vi "10-Tap 8-Bit Camera with DRAM (Host) - calibration.vi"() -> ()   [LabVIEW 2018]
doc: "This is the host VI for the 10-Tap 8-Bit Camera with DRAM example. This example demonstrates how to acquire images from a 10-tap, 8-bit, extended configuration, Camera Link camera and display the images on the host. This example supports area scan and line scan cameras for both continuous and finite acquisitions.\n\nThis example also demonstrates the use of DRAM as a frame buffer for very high speed acquisitions. Data packing and flow-control are also employed to maximize use of the available DRAM and FIFOs in terms of both memory space and performance.\n\nAdditionally, the example demonstrates the serial server, which allows third-party camera configuration utilities to communicate with the camera using the Camera Link serial interface while this VI is running."
uses:
  <vilib>/userdefined/High Color/nirio_resource_hc.ctl
  <vilib>/Analysis/Matrix/Datatypes/RealMatrix.ctl
  <vilib>/Platform/TimedLoop/XDataNode/timing_clust.ctl
  <vilib>/Platform/TimedLoop/XDataNode/nitl_modes.ctl
  <vilib>/Platform/TimedLoop/XDataNode/wakeup.ctl
  <vilib>/DAQmx/write.llb/DAQmx Write (Analog DBL 1Chan 1Samp).vi
  <vilib>/Analysis/baseanly.llb/Real A x B.vi
  <vilib>/FPGAPlugInAG/PCIe-1473R/niLvFpga_Open_PCIe-1473R.vi
  <vilib>/rvi/interface/common/dynamic/niFpgaDynamicAddResources.vi
  <vilib>/FPGAPlugInAG/Dynamic/niLvFpga_Reset_Dynamic.vi
  <vilib>/Analysis/Matrix/Numeric/Conversions/Array To Matrix - RA2.vi
  <userlib>/DAQNavi Polymorphic VI/create/DAQNavi Create Channel(CI-UpDown Count Value).vi
  <vilib>/Utility/error.llb/Error Cluster From Error Code.vi
  <vilib>/rvi/errors/niLvFpgaAdjustHostInterfaceError.vi
  <vilib>/FPGAPlugInAG/Dynamic/niLvFpga_Run_Dynamic.vi
  <vilib>/rvi/interface/common/niFpgaWaitOnOcc.vi
  <userlib>/DAQNavi Polymorphic VI/read/DAQNavi Read (Counter Count Value 1Chan 1Samp).vi
  <vilib>/Analysis/Matrix/Numeric/Conversions/Array To Matrix - RA.vi
  <vilib>/Analysis/Matrix/Numeric/Conversions/Matrix To Array - RM.vi
  <vilib>/DAQmx/miscellaneous.llb/DAQmx Fill In Error Info.vi
  <vilib>/FPGAPlugInAG/Dynamic/niLvFpga_Close_Dynamic.vi
  <vilib>/platform/TimedLoop/XDataNode/XDataNode.xnode
  <vilib>/rvi/interface/nirviOpenFPGA/nirviOpenFPGA.xnode
  FPGA Bitfiles/10-Tap8-bitCamer_FPGATarget_10-Tap8-bitCamer_C490DC32.lvbitx
  <vilib>/rvi/interface/nirviMethod/nirviMethod.xnode
  <vilib>/ErrorRing/Error Ring.xnode
  <vilib>/rvi/interface/nirviReadWriteControl/nirviReadWriteControl.xnode
  <vilib>/rvi/interface/nirviCloseFPGA/nirviCloseFPGA.xnode
  <vilib>/rvi/interface/Simulation/niFpgaSimulationCallBeginRW.vi
  <vilib>/rvi/errors/niLvFpgaMergeErrorWithErrorCode.vi
  NiFpgaLv.dll
  <vilib>/FPGAPlugInAG/Dynamic/niLvFpga_ConfigureFifo_Dynamic.vi
  <vilib>/FPGAPlugInAG/Dynamic/niLvFpga_StartFifo_Dynamic.vi
  <vilib>/FPGAPlugInAG/Dynamic/niLvFpga_ReadFifo_Dynamic.vi
  <vilib>/Platform/TimedLoop/XDataNode/XDNodeRunTimeDep.lvlib
  <resource>/objmgr/ni.dex.rc
  MPC_dll_4_vs17_cv3_4/x64/Release/MPC_dll_4_vs17_cv3_4.dll
  fish tracking dll vc17 opencv3_4/x64/Release/fish tracking dll vc17 opencv3_4.dll
  <vilib>/Analysis/NI_AALBase.lvlib
  <vilib>/Analysis/Matrix/NI_Matrix.lvlib
panel:
  out "Cluster":cluster{"data":i32, i32}
  out "Real Matrix 5":T1
  out "Real Matrix 4":T1
  out "Real Matrix 2":T1
  out "Real Matrix":T1
  out "A x B 2":T1
  out "A x B":T1
  out "error out":errorcluster
  in  "send":bool
  out "Is Connected":bool
  in  "update ratio":dbl
  in  "Start Serial Server":bool=TRUE
  in  "Stopped 2":bool
  in  "display":bool=TRUE
  out "Image":T2(plugin-control)
  in  "reset 2":bool
  in  "reset frame":bool
  in  "reset position":bool
  out "max load a frame":dbl
  out "max load a position":dbl
  out "# elements in queue":i32
  out "element":dbl[](array[numeric])
  in  "start sending":bool
  out "connected":bool
  in  "Acquire":bool
  out "max distance 2":i32
  out "out of FOV 2":i32
  in  "count":bool
  out "max distance":i32
  out "out of FOV":i32
  out "Stage Position Y":i32=520
  out "Stage Position X":i32=520
  out "#timeout3":i32
  out "#timeout1":i32
  out "max time4 image and position loading":dbl
  out "max time3 total":dbl
  out "max time2 detection":dbl
  out "max time1 detection+command":dbl
  out "time loading a frame":dbl
  in  "length of fish_history":i32=4
  in  "m(length of kernel)":i32=30
  out "Heading":cluster{dbl, dbl}
  out "BKG_Global":T2(plugin-control)
  out "process":i32
  in  "Target Y":i32(slide)=171 min=0 max=384 scale=130.0..230.0
  in  "Target X":i32(slide)=179 min=0 max=520 scale=130.0..230.0
  out "y":dbl
  out "x":dbl
  in  "Controller":picture
  out "Y Resolution":i32
  out "X Resolution":i32
  in  "Track":bool
  out "Frame #":i32=72
  out "电压2":dbl
  out "电压1":dbl
  out "fish FOUND":bool
  out "Centroid":cluster{"x":i32, "y":i32}
  out "TimeDelay":dbl
  in  "DMA Buffer Size\n(In Images)":u32=64 caption="DMA Buffer Size"
  in  "Signal Mapping":T3(ring)=enum."Basler 10-tap"
  out "Acq In Progress":bool
  in  "Line Scan":bool
  in  "Cancel":bool
  out "Acq'd Frame Width":u32
  in  "Stopped":bool
  in  "RIO Device":T4="RIO0"
  out "DMA Write Timeout":bool
  out "Frames Acq'd":u32
  out "Acq'd Frame Height":u32
  in  "Stop":bool
  in  "Image Height":u32=360 max=65535
  in  "Image Width":u32=360 max=65535 step=40
  out "Initialized":bool
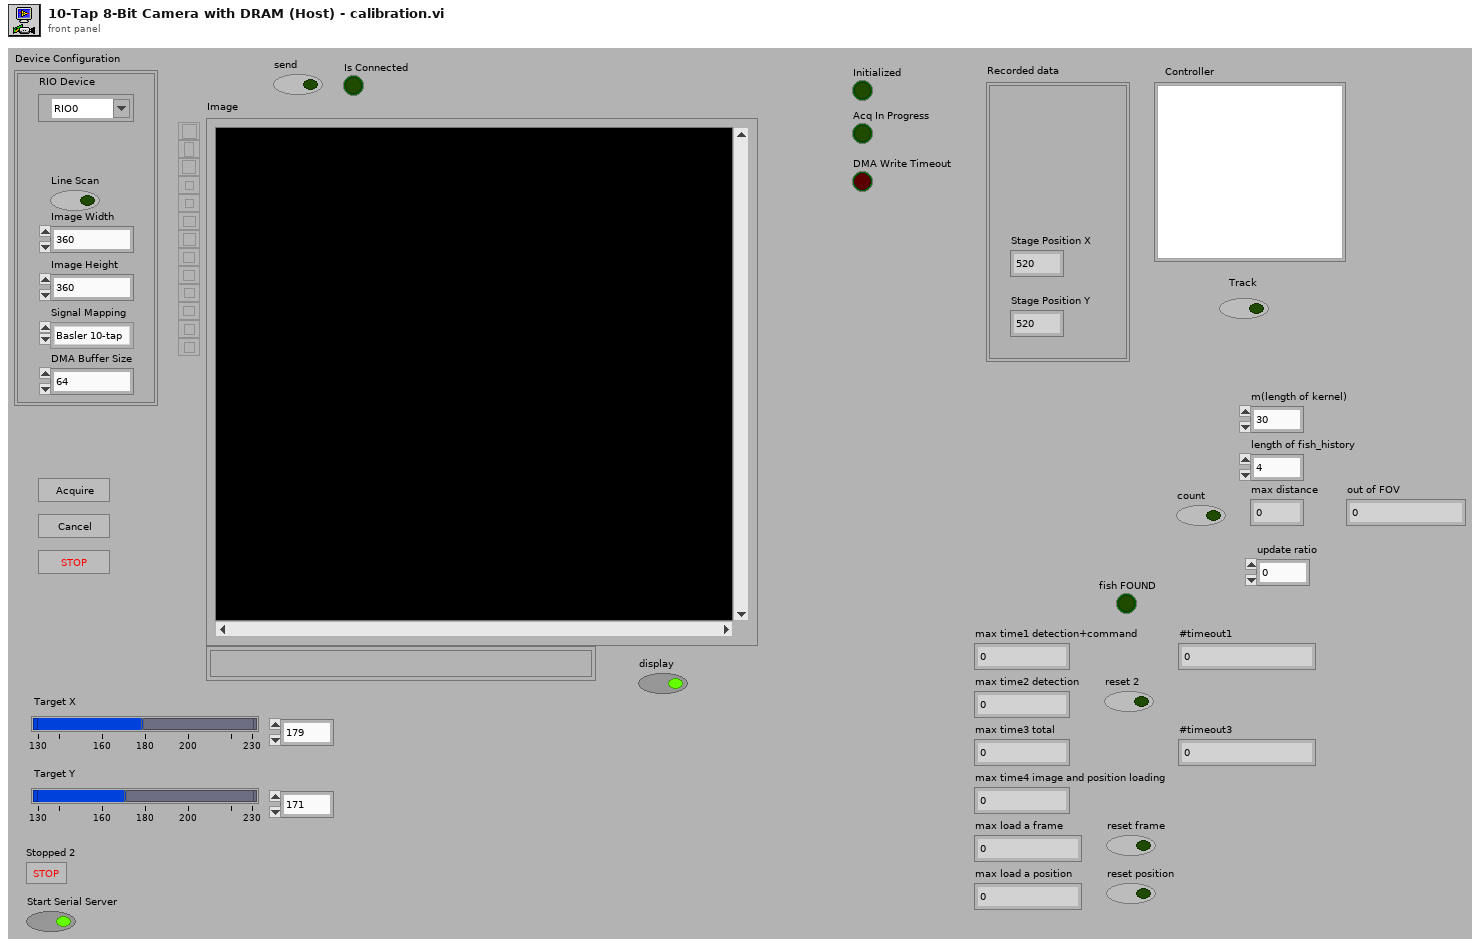
[diagram p1: front panel]
types:
  T1 = typedef "NI_Matrix.lvlib/RealMatrix.ctl" = dbl[][]
  T2 = typedef "IMAQ Image.ctl" = refnum<image>
  T3 = enum8{"Standard", "Basler 10-tap", "Vosskühler 10-tap"}
  T4 = typedef "nirio_resource_hc.ctl" = tag
  T5 = typedef "Image Type" = u32
  T6 = typedef "XDNodeRunTimeDep.lvlib/timing_clust.ctl" = cluster{"Expected End [f-1]":u64, "Actual End [f-1]":u64, "Finished Late? [f-1]":bool, "Expected End [i-1]":u64, "Actual End [i-1]":u64, "Finished Late? [i-1]":bool, "Expected Start [i]":u64, "Actual Start [i]":u64, "Expected Start [f]":u64, "Actual Start [f]":u64, "Source Name":string, "Structure Name":string, "Period":i64, "Deadline":i64, "Offset":i64, "Start":i64, "Priority":i32, "Timeout":i32, "Mode":T7, "Wakeup Reason":T8, "Error":errorcluster, "Source Type":string, "Secondary Source Type":string, "Global End Time":u64, "Global Start Time":u64, "Frame Duration":u64, "Iteration Duration":u64, "Assigned CPU":i32, "I/O Scan Engine Mode":u32}
  T7 = typedef "XDNodeRunTimeDep.lvlib/nitl_modes.ctl" = enum32{"No Change", "Process missed periods, maintain original phase", "Discard missed periods, maintain original phase", "Process missed periods, ignore original phase", "Discard missed periods, ignore original phase"}
  T8 = typedef "XDNodeRunTimeDep.lvlib/wakeup.ctl" = enum32{"Normal", "Aborted", "Asynchronous wakeup", "Timing source error", "Timed loop error", "Timeout"}
  T9 = enum16{"big-endian, network order", "native, host order", "little-endian"}
  T10 = enum32{"Map Pixel Pointer", "Unmap Pixel Pointer", "Get Pixels Infos"}
  T11 = typedef "LVPoint32TypeDef.ctl" = cluster{"Horizontal":i32, "Vertical":i32}
  T12 = typedef "LVPositionTypeDef.ctl" = cluster{"Left":i32, "Top":i32}
  T13 = typedef "LVBoundsTypeDef.ctl" = cluster{"Width":u32, "Height":u32}
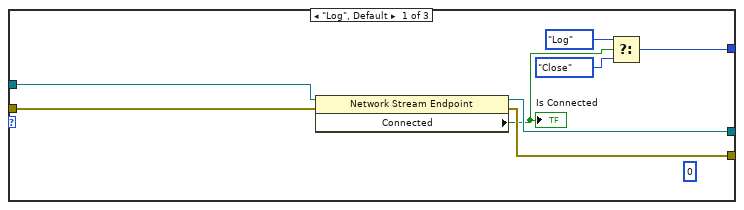
[diagram p4: hidden frame]
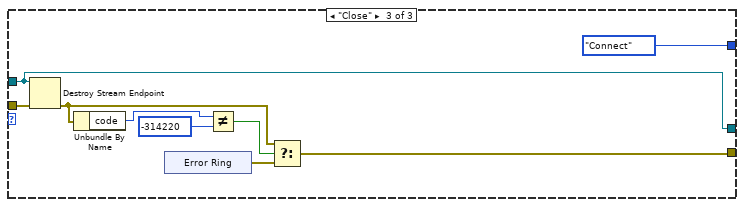
[diagram p5: hidden frame]
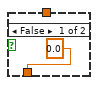
[diagram p12: hidden frame]
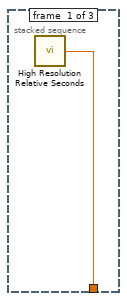
[diagram p13: hidden frame]
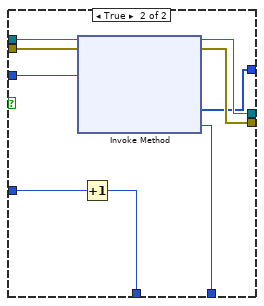
[diagram p14: hidden frame]
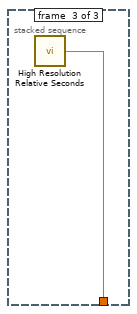
[diagram p15: hidden frame]
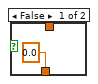
[diagram p16: hidden frame]
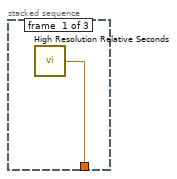
[diagram p17: hidden frame]
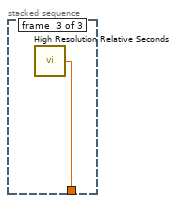
[diagram p18: hidden frame]
diagram:
  w23 = 72 ("n_templates")
  w25 = 0
  w46 = 2
  w40 = 0
  w47 = 0.0
  w72 = T5 0 items=["Grayscale (U8)", "Grayscale (I16)", "Grayscale (SGL)", "Complex (CSG)", "RGB (U32)", "HSL (U32)", "RGB (U64)", "Grayscale (U16)"] ("Image Type")
  w86 = refnum<k21> "Stage_Y"  # DAQmx任务名
  w87 = refnum<k21> "Stage_X"  # DAQmx任务名
  w89 = T5 0 items=["Grayscale (U8)", "Grayscale (I16)", "Grayscale (SGL)", "Complex (CSG)", "RGB (U32)", "HSL (U32)", "RGB (U64)", "Grayscale (U16)"] ("Image Type")
  w95 = u32 8  # Pixels per DMA word
  w126 = T5 0 items=["Grayscale (U8)", "Grayscale (I16)", "Grayscale (SGL)", "Complex (CSG)", "RGB (U32)", "HSL (U32)", "RGB (U64)", "Grayscale (U16)"] ("Image Type")
  # "Start the Serial Server to allow serial communication\nwith the camera. This allows third-party camera\nconfiguration utilites to be used."
  # "If your camera outputs active-low enable\nsignals or does not use DVAL then you \ncan change the configuration here."
  # "Configure the DMA FIFO memory buffer to be\nlarge enough for several frames. This provides\nbuffering to help deal with system latencies."
  # "Start running\nthe FPGA VI."
  # "Reset FPGA to clear\nany current state."
  # "Read the specified image\nwidth and height. In this\nexample, these must be set\nbefore starting the VI."
  # "Merge any errors.\nClean up the image.\nClose the FPGA reference.\nDisplay any errors."
  # "Acquire frames as requested.\nUse the width and height to determine how much data to read from the DMA FIFO.\nConvert the data into a Vision Image for display."
  # "Monitor the acquisition status"
  # "Create an image of the type to be displayed."
  # "Initialize the acquisition interface on the FPGA.  This will\nwait until a pixel clock is detected from the camera."
  # "Initialize the DMA FIFO for transferring\ndata from FPGA target to the host."
  # "Configure the Camera Link interface.\nThis needs to be done prior to running\nthe FPGA block diagram."
  # "Open a reference to the FPGA bitstream\nand initialize the user interface."
  n1 = flat-sequence {
    tunnel: [w132] -> w121
    tunnel: [w131] -> w130
    frame #0 {
      w135 = u32 0 ("Num Lines Acq'd")
      w134 = FALSE ("stop")
      n2 = local write "DMA Write Timeout"(w134) -> ()
      n3 = local write "Acq'd Frame Width"(w135) -> ()
      n4 = local write "Acq'd Frame Height"(w135) -> ()
      n5 = local write "Stopped"(w134) -> ()
      n6 = local write "Frames Acq'd"(w135) -> ()
      n7 = local write "Initialized"(w134) -> ()
      n8 = xnode "打开FPGA VI引用句柄"("resource name"="RIO Device") -> ("FPGA VI Reference Out"=w132:refnum<k20>, "error out"=w131:errorcluster)  [unwired: 1 in]
    }
  }
  n9 = xnode "Invoke Method"("FPGA VI Reference In"=w121, "error in"=w130) -> ("FPGA VI Reference Out"=w111:refnum<k20>, "error out"=w113:errorcluster)
  n10 = xnode "Read/Write Control"("FPGA VI Reference In"=w111, "error in"=w113, "CL Config.FVAL Active High"=TRUE ("IO Module Config.CL FVAL Active High"), "CL Config.LVAL Active High"=TRUE ("IO Module Config.CL LVAL Active High"), "CL Config.DVAL Active High"=TRUE ("IO Module Config.CL DVAL Active High"), "CL Config.Spare Active High"=TRUE ("IO Module Config.CL Spare Active High"), "CL Config.Line Scan"="Line Scan", "Acq Control.Ignore DVAL"=FALSE ("CL Config.Line Scan"), "CL Config.Configuration"=enum8{"Base", "Medium", "Full"}."Full", "CL Config.Signal Mapping"="Signal Mapping") -> ("FPGA VI Reference Out"=w114:refnum<k20>, "error out"=w112:errorcluster)
  n11 = xnode "Invoke Method"("FPGA VI Reference In"=w114, "error in"=w112) -> ("FPGA VI Reference Out"=w92:refnum<k20>, "error out"=w91:errorcluster)  [unwired: 1 in]
  n12 = Multiply(x="Image Height", y="Image Width") -> (x*y=w94:u32)
  n13 = Quotient & Remainder(x=w94, y=w95) -> (floor(x/y)=w93:u32)  [unwired: 1 out]
  n14 = Multiply(x=w93, y="DMA Buffer Size\n(In Images)") -> (x*y=w105:u32)
  n15 = xnode "Invoke Method"("FPGA VI Reference In"=w92, "error in"=w91, "请求的深度"=w105) -> ("FPGA VI Reference Out"=w120:refnum<k20>, "error out"=w119:errorcluster)  [unwired: 1 out]
  n16 = xnode "Invoke Method"("FPGA VI Reference In"=w120, "error in"=w119) -> ("FPGA VI Reference Out"=w106:refnum<k20>, "error out"=w118:errorcluster)
  n17 = xnode "读取/写入控件"("FPGA VI Reference In"=w106, "error in"=w118, "Acq Control.Initialize"=TRUE ("Arm Acquisition")) -> ("FPGA VI Reference Out"=w129:refnum<k20>, "error out"=w128:errorcluster)
  n18 = while {
    tunnel: w129 -> [w143]
    tunnel: w128 -> [w142]
    tunnel: [w141] -> w10
    tunnel: [w145] -> w102
    i -> [w137]
    stop <- w148 stop-if-true
    # "A custom error is generated if the acquisition unit has not become\ninitialized within 2 seconds. This typically occurs when a camera is\nnot connected, is not powered, or is not of the correct type."
    n19 = xnode "读取/写入控件"("FPGA VI Reference In"=w143, "error in"=w142) -> ("FPGA VI Reference Out"=w141:refnum<k20>, "error out"=w140:errorcluster, "Acq Status.Initialized"=w139:bool)
    n20 = Wait (ms)(milliseconds to wait=u32 100) -> ()  [unwired: 1 out]
    n21 = Greater?(x=w137, y=20) -> (0:w138:bool)
    n22 = case shown="True" w138 {
      tunnel: [w150 FALSE] -> w144
      tunnel: w139 -> [w150 _]
      tunnel: w140 -> [w149 w152]
      tunnel: [w149 w154] -> w145
      frame False {
      }
      frame True {
        n23 = Merge Errors(w152, errorcluster {"status"=TRUE, "code"=-8999, "source"="Acquisition Initialization: This error typically occurs when a camera is not properly connected, is not powered, or is not of the correct type."} ("error in")) -> (w154:errorcluster)
      }
    }
    "Initialized" <- w144
    n24 = Unbundle By Name(w145) -> ("status"=w147:bool)
    n25 = Or(x=w147, y=w144) -> (x .or. y?=w148:bool)
  }
  n26 = case shown="True" "Start Serial Server" {
    tunnel: [_ w155] -> w9
    tunnel: w10 -> [_ w156]
    frame False {
    }
    frame True {
      n27 = control-ref of="Stopped 2"() -> (w157:refnum<vi>)
      n28 = call "SerialServer.vi"("Stop Refnum"=w157, "FPGA VI Reference In"=w156) -> ("FPGA VI Reference Out"=w155:refnum<k20>)  [unwired: 5 in]
    }
  }
  n29 = call "IMAQ Create"("Image Name"="Image", "Image Type"=w126, "error in (no error)"=w102) -> ("New Image"=w99:T2, "error out"=w98:errorcluster)  [unwired: 2 in]
  n30 = Add(x="length of fish_history", y=1) -> (x+y=w42:i32)
  n31 = Initialize Array(0.0, 7) -> (w12:dbl[])
  n32 = Obtain Queue(max queue size (-1, unlimited)=3, name (unnamed)="tracking result" ("Image Name"), element data type=w12) -> (queue out=w8:refnum<queue>)  [unwired: 2 in, 2 out]
  n33 = Multiply(x=w46, y=w42) -> (x*y=w39:i32)
  n34 = To Unsigned Byte Integer(number=w25) -> (unsigned 8bit integer=w26:u8)
  n35 = Add(x="m(length of kernel)", y=1) -> (x+y=w27:i32)
  n36 = Initialize Array(w26, w25, w25, w25) -> (w24:u8[][][])
  n37 = for {
    N: w23 -> [_]
    shift-right: [w159] -> w22
    shift-left: w24 -> [w160]
    i -> [w158]
    w164 = T5 0 items=["Grayscale (U8)", "Grayscale (I16)", "Grayscale (SGL)", "Complex (CSG)", "RGB (U32)", "HSL (U32)", "RGB (U64)", "Grayscale (U16)"] ("Image Type")
    n38 = Number To Decimal String(number=w158) -> (decimal integer string=w168:string)  [unwired: 1 in]
    n39 = Concatenate Strings(w168, ".jpg") -> (w167:string)
    n40 = Build Path(base path=path "F:/TrackingUsingOpenCV3_with_bkg_subtr_and_pred_and_temp_matching_nodisplay - 210309/templates" ("Templates Path"), name or relative path=w167) -> (appended path=w166:path)
    n41 = call "IMAQ Create"("Image Name"="Temp", "Image Type"=w164) -> ("New Image"=w163:T2)  [unwired: 3 in, 1 out]
    n42 = call "IMAQ ReadFile"("File Path"=w166, "Image"=w163) -> ("Image Out"=w162:T2)  [unwired: 5 in, 4 out]
    n43 = call "IMAQ ImageToArray"("Image"=w162) -> ("Image Pixels (U8)"=w161:u8[][])  [unwired: 3 in, 4 out]
    n44 = Insert Into Array(array=w160, index (dim 0)=w158, new element=w161) -> (w159:u8[][][])  [unwired: 2 in]
  }
  n45 = Multiply(x=w46, y=w27) -> (x*y=w45:i32)
  n46 = Obtain Queue(max queue size (-1, unlimited)=w45, name (unnamed)="command_history", element data type=w47) -> (queue out=w49:refnum<queue>)  [unwired: 2 in, 2 out]
  n47 = Obtain Queue(max queue size (-1, unlimited)=w39, name (unnamed)="stage_position_history", element data type=w40) -> (queue out=w38:refnum<queue>)  [unwired: 2 in, 2 out]
  n48 = Obtain Queue(max queue size (-1, unlimited)=w39, name (unnamed)="fish_tr_history", element data type=w40) -> (queue out=w51:refnum<queue>)  [unwired: 2 in, 2 out]
  n49 = Obtain Queue(max queue size (-1, unlimited)=w39, name (unnamed)="fish_heading_history", element data type=w47) -> (queue out=w50:refnum<queue>)  [unwired: 2 in, 2 out]
  n50 = for "For循环" {
    N: w45 -> [_]
    tunnel: w49 -> [w173]
    tunnel: [w172] -> w48
    n51 = Lossy Enqueue Element(queue=w173, element=0.0) -> (queue out=w172:refnum<queue>)  [unwired: 1 in, 3 out]
  }
  n52 = call-poly <userlib>:"DAQNavi Create Channel.vi"("physical channels"="PCI-1784,BID#1/cntr0" ("Image Name"), "signal counting type"="AbPhaseX4" ("Image Name"), "initial value"="0" ("Image Name")) -> ("task out"=w66:i32)  [unwired: 11 in, 1 out]
  n53 = call-poly <userlib>:"DAQNavi Create Channel.vi"("physical channels"="PCI-1784,BID#1/cntr1" ("Image Name"), "signal counting type"="AbPhaseX4" ("Image Name"), "initial value"="0" ("Image Name")) -> ("task out"=w65:i32)  [unwired: 11 in, 1 out]
  n54 = call "IMAQ Create"("Image Name"="BkgImageOpenCV", "Image Type"=w72) -> ("New Image"=w74:T2)  [unwired: 3 in, 1 out]
  n55 = call <userlib>:"DAQNavi Start Task.vi"("task in"=w66) -> ("task out"=w62:i32)  [unwired: 9 in, 1 out]
  n56 = call <userlib>:"DAQNavi Start Task.vi"("task in"=w65) -> ("task out"=w61:i32)  [unwired: 9 in, 1 out]
  n57 = while "Target->Host Data Writer" {
    shift-right: [w181] -> w2
    shift-left: _ -> [w184]
    shift-right: [w180] -> _
    shift-left: _ -> [w185]
    shift-right: [w182] -> _
    shift-left: enum16{"Log", "Connect", "Close"}."Log" -> [w183]
    tunnel: w8 -> [w176]
    tunnel: [w175] -> w1
    stop <- w174 stop-if-true
    # "Send Data to Host VI"
    n58 = case shown="\"Connect\"" w183 {
      tunnel: [w202 w209 w227] -> w180
      tunnel: w185 -> [w205 _ w227]
      tunnel: w184 -> [w204 _ w228]
      tunnel: [w203 w210 w221] -> w181
      tunnel: [w206 enum16{"Log", "Connect", "Close"}."Log" enum16{"Log", "Connect", "Close"}."Connect"] -> w182
      frame "Log", Default {
        (unwired) 0 ("timeout ms")
        n59 = property class="Network Stream Endpoint"(reference=w205, error in=w204) -> (reference out=w202:refnum<k21>, error out=w203:errorcluster, "Connected"=w201:bool)
        "Is Connected" <- w201
        n60 = Select(t=enum16{"Log", "Connect", "Close"}."Log", s=w201, f=enum16{"Log", "Connect", "Close"}."Close") -> (s? t:f=w206:enum16{"Log", "Connect", "Close"})
      }
      frame "Connect" {
        n61 = Concatenate Strings("//" ("reader url"), "192.168.1.30" ("Target IP Address")) -> (w215:string)
        n62 = Concatenate Strings(w215, "/reader1" ("reader url")) -> (w213:string)
        n63 = Create Network Stream Writer Endpoint(5:-1 ("timeout in ms (-1)"), 7:70, 9:0.0, 10:w213, 11:"writer") -> (0:w210:errorcluster, 3:w209:refnum<k21>)  [unwired: 2 in]
      }
      frame "Close" {
        n64 = Destroy Stream Endpoint(8:w228, 11:w227) -> (0:w222:errorcluster)
        n65 = Unbundle By Name(w222) -> ("code"=w226:i32)
        n66 = xnode "Error Ring"() -> ("error out"=w223:errorcluster)
        n67 = Not Equal?(x=w226, y=-314220) -> (x != y?=w224:bool)
        n68 = Select(t=w222, s=w224, f=w223) -> (s? t:f=w221:errorcluster)
      }
    }
    n69 = property class="Network Stream Endpoint"(reference=w180, error in=w181) -> (reference out=w178:refnum<k21>, error out=w177:errorcluster, "Connected"=w179:bool)
    n70 = case shown="True" w179 {
      tunnel: w178 -> [_ w190]
      tunnel: w177 -> [_ w191]
      tunnel: w176 -> [w186 w189]
      tunnel: [w186 w187] -> w175
      frame False {
      }
      frame True {
        n71 = Get Queue Status(queue=w189) -> (queue out=w193:refnum<queue>)  [unwired: 2 in, 7 out]
        n72 = Dequeue Element(queue=w193) -> (queue out=w187:refnum<queue>, element=w192:dbl[])  [unwired: 2 in, 2 out]
        n73 = case shown="True" "send" {
          tunnel: w192 -> [_ w198]
          tunnel: w191 -> [_ w197]
          tunnel: w190 -> [_ w196]
          frame False {
          }
          frame True {
            w199 = 0 ("timeout ms (-1)")
            n74 = shared-variable-write(w196, w197, w198, w199) -> (w195:refnum<k21>, w200:errorcluster)  [unwired: 1 out]
            n75 = Flush Stream(8:w200, 9:w199, 11:w195) -> (0:→"error out":errorcluster)  [unwired: 1 in, 2 out]
          }
        }
      }
    }
    n76 = local read "Stop"() -> (w174:bool)
  }
  n77 = disable-structure shown="Disabled" {
    disable-tunnel: w8 -> [w231 _]
    frame Disabled {
      n78 = Concatenate Strings("//" ("reader url"), "192.168.1.19" ("Target IP Address")) -> (w242:string)
      n79 = Concatenate Strings(w242, "/reader1" ("reader url")) -> (w240:string)
      n80 = Create Network Stream Writer Endpoint(7:70, 9:0.0, 10:w240, 11:"writer") -> (0:w245:errorcluster, 3:w247:refnum<k21>)  [unwired: 3 in]
      n81 = property class="Network Stream Endpoint"(reference=w247, error in=w245) -> (reference out=w238:refnum<k21>, error out=w237:errorcluster, "Connected"=→"connected":bool)
      n82 = node-c288() -> (w251:T6)  [unwired: 4 in]
      n83 = timed-loop {
        tunnel: w231 -> [w258]
        tunnel: w238 -> [w257]
        tunnel: w237 -> [w256]
        tunnel: [w255] -> w234
        tunnel: [w254] -> w233
        tunnel: [w253] -> w232
        timing: w251 -> [_]
        timing-out: [_] -> w250
        stop <- w252 stop-if-true
        n84 = node-c288() -> ()  [unwired: 1 in, 1 out]
        n85 = case shown="True" "start sending" {
          tunnel: w257 -> [w263 w276]
          tunnel: w256 -> [w262 w275]
          tunnel: w258 -> [w264 w266]
          tunnel: [w264 w274] -> w255
          tunnel: [w263 w269] -> w254
          tunnel: [w262 w268] -> w253
          frame False {
          }
          frame True {
            w270 = 0
            n86 = Get Queue Status(queue=w266) -> (queue out=w267:refnum<queue>, # elements in queue=w265:i32)  [unwired: 2 in, 6 out]
            n87 = disable-structure shown="Disabled" {
              disable-tunnel: w265 -> [w277 _]
              frame Disabled {
                "# elements in queue" <- w277
              }
              frame Enabled {
              }
            }
            n88 = Dequeue Element(queue=w267) -> (queue out=w274:refnum<queue>, element=w273:dbl[])  [unwired: 2 in, 2 out]
            n89 = disable-structure shown="Disabled" {
              disable-tunnel: w273 -> [w278 _]
              frame Disabled {
                "element" <- w278
              }
              frame Enabled {
              }
            }
            n90 = shared-variable-write(w276, w275, w273, w270) -> (w272:refnum<k21>, w271:errorcluster)  [unwired: 1 out]
            n91 = Flush Stream(8:w271, 9:w270, 11:w272) -> (0:w268:errorcluster, 3:w269:refnum<k21>)  [unwired: 1 in, 1 out]
          }
        }
        n92 = local read "Stop"() -> (w252:bool)
        n93 = node-c288() -> ()  [unwired: 1 in, 1 out]
      }
      n94 = node-c288(w250) -> ()  [unwired: 1 out]
      n95 = Release Queue(queue=w234) -> ()  [unwired: 2 in, 3 out]
      n96 = Flush Stream(8:w232, 11:w233) -> (0:w235:errorcluster, 3:w236:refnum<k21>)  [unwired: 2 in, 1 out]
      n97 = Destroy Stream Endpoint(8:w235, 11:w236) -> ()  [unwired: 1 out]
    }
    frame Enabled {
    }
  }
  n98 = call-poly <vilib>:"Array To Matrix.vi"("Real 2D Array"=dbl[][] [[1.506559, -0.036078], [0.030048, 1.495542]]) -> ("Real Matrix"=w4:T1)
  "Real Matrix 5" <- w4
  n99 = call "IMAQ ReadFile"("File Path"=path "F:/TrackingUsingOpenCV3_with_bkg_subtr_and_pred_and_temp_matching_nodisplay/fish tracking dll vc17 opencv3_4/bkg_global.png" ("Bkg Image Path"), "Image"=w74) -> ("Image Out"=w71:T2)  [unwired: 5 in, 4 out]
  n100 = call-poly <vilib>:"Array To Matrix.vi"("Real 2D Array"=dbl[][] [[1.506559, -0.036078, 0.0], [0.030048, 1.495542, 1.506559], [-12.463135, -1.547689, 1.0]]) -> ("Real Matrix"=w5:T1)
  "Real Matrix 4" <- w5
  n101 = node-c288() -> (w17:T6)  [unwired: 4 in]
  n102 = call "IMAQ Create"("Image Name"="DstImageOpenCV", "Image Type"=w89) -> ("New Image"=w88:T2)  [unwired: 3 in, 1 out]
  n103 = while {
    tunnel: w10 -> [w291]
    tunnel: [w294] -> w115
    stop <- w293 stop-if-true
    w284 = u32 10  # Pixels per clock
    # "Update status indicators"
    n104 = Wait Until Next ms Multiple(millisecond multiple=u32 100) -> ()  [unwired: 1 out]
    n105 = xnode "Read/Write Control"("FPGA VI Reference In"=w291) -> ("error out"=w290:errorcluster, "Acq Status.Lines Per Frame"=w287:u32, "Acq Status.Frames Acq'd"=w289:u32, "Acq Status.Clocks Per Line"=w285:u32, "Acq Status.Acq In Progress"=→"Acq In Progress":bool, "Acq Status.DMA Write Timeout"=w282:bool)  [unwired: 1 in, 1 out]
    "DMA Write Timeout" <- w282
    n106 = Multiply(x=w285, y=w284) -> (x*y=w286:u32)
    n107 = disable-structure shown="Disabled" {
      disable-tunnel: w289 -> [w297 _]
      disable-tunnel: w287 -> [w296 _]
      disable-tunnel: w286 -> [w295 _]
      frame Disabled {
        "Acq'd Frame Height" <- w296
        "Frames Acq'd" <- w297
        "Acq'd Frame Width" <- w295
      }
      frame Enabled {
      }
    }
    n108 = local read "Stopped"() -> (w281:bool)
    n109 = Compound Arithmetic op=AND(w282, invert w281) -> (w283:bool)
    n110 = case shown="True" w283 {
      tunnel: w290 -> [w302 _]
      tunnel: [w302 errorcluster {"status"=TRUE, "code"=-8999, "source"="DMA Write Timeout: The write operation to the DMA FIFO on the FPGA timed out. This can be caused by the DMA FIFO not being started or the DMA FIFO overflowing. Make sure that Start is being called on the DMA FIFO. Also make sure that the host application is reading from the DMA FIFO fast enough to prevent it from overflowing."} ("error out")] -> w294
      frame False {
      }
      frame True {
      }
    }
    n111 = flat-sequence {
      tunnel: w294 -> [w301]
      tunnel: [w299] -> w293
      frame #0 {
        n112 = Unbundle By Name(w301) -> ("status"=w300:bool)
        n113 = Or(x=w300, y="Stopped") -> (x .or. y?=w299:bool)
        n114 = local write "Stopped"(w299) -> ()
      }
    }
  }
  n115 = call <vilib>:"Simple Error Handler.vi"("error in (no error)"=w2) -> ()  [unwired: 4 in, 5 out]
  n116 = Release Queue(queue=w1) -> ()  [unwired: 2 in, 3 out]
  n117 = Open/Create/Replace File(file path (use dialog)=path "E:/Time.txt" ("Folder"), operation (0:open)=4) -> (refnum out=w31:refnum<file>)  [unwired: 4 in, 2 out]
  n118 = call <vilib>:"DAQmx Start Task.vi"("task/channels in"=w86) -> ("task out"=w84:refnum<k21>)  [unwired: 13 in, 1 out]
  n119 = call <vilib>:"DAQmx Start Task.vi"("task/channels in"=w87) -> ("task out"=w85:refnum<k21>)  [unwired: 13 in, 1 out]
  n120 = timed-loop {
    tunnel: w10 -> [w427]
    tunnel: w98 -> [w426]
    tunnel: w93 -> [w323]
    tunnel: "Image Height" -> [w322]
    tunnel: "Image Width" -> [w431]
    tunnel: w99 -> [w430]
    tunnel: [w312] -> w116
    tunnel: [w429] -> w125
    tunnel: [w428] -> w123
    tunnel: w88 -> [w425]
    tunnel: w85 -> [w424]
    tunnel: w84 -> [w423]
    tunnel: [w422] -> w83
    tunnel: [w421] -> w82
    tunnel: w71 -> [w420]
    tunnel: w62 -> [w413]
    tunnel: w61 -> [w412]
    tunnel: [w411] -> w58
    tunnel: [w410] -> w57
    shift-right: [w416] -> _
    shift-left: u32 0 -> [w417]
    shift-right: [w414] -> _
    shift-left: cluster{"y":i32, "x":i32} {"y"=0, "x"=0} ("Centroid") -> [w415]
    tunnel: w48 -> [w409]
    tunnel: w51 -> [w408]
    tunnel: w50 -> [w407]
    tunnel: w38 -> [w406]
    tunnel: [w405] -> w37
    tunnel: [w404] -> w36
    tunnel: [w403] -> w35
    tunnel: [w402] -> w34
    tunnel: w31 -> [w400]
    tunnel: [w399] -> w30
    shift-right: [w398] -> _
    shift-left: _ -> [w397]
    tunnel: w23 -> [w396]
    tunnel: w22 -> [w395]
    tunnel: w8 -> [w394]
    timing: w17 -> [_]
    timing-out: [_] -> w16
    border: u32 0 -> [_]
    tunnel: w5 -> [w308]
    tunnel: w4 -> [w306]
    i -> [w401]
    stop <- w418 stop-if-true
    # "Read one frame\nfrom DMA FIFO"
    # "If we're in an acquisition, wait until\nwe have at least one frame to read."
    n121 = node-c288() -> ()  [unwired: 1 in, 1 out]
    n122 = stacked-sequence {
      tunnel: [_ w442 _] -> w429
      tunnel: w427 -> [_ w441 _]
      tunnel: w426 -> [_ w440 _]
      tunnel: [_ w439 _] -> w312
      tunnel: [_ w438 _] -> w393
      tunnel: w323 -> [_ w437 _]
      tunnel: w322 -> [_ w436 _]
      tunnel: [w435 _ _] -> w320
      tunnel: [_ _ w490] -> w321
      frame #0 {
        n123 = call <vilib>:"High Resolution Relative Seconds.vi"() -> ("relative seconds"=w435:dbl)
      }
      frame #1 {
        n124 = while {
          tunnel: [w448] -> w438
          tunnel: w437 -> [w445]
          shift-right: [w456] -> w442
          shift-left: w441 -> [w455]
          shift-right: [w449] -> w439
          shift-left: w440 -> [w454]
          tunnel: w436 -> [w443]
          stop <- w444 stop-if-true
          n125 = feedback #1() -> (w450:u32)
          n126 = while {
            tunnel: w455 -> [w486]
            tunnel: w454 -> [w485]
            tunnel: [w483] -> w453
            tunnel: [w484] -> w452
            tunnel: w450 -> [w489]
            tunnel: [w487] -> w446
            stop <- w488 stop-if-true
            n127 = xnode "Read/Write Control"("FPGA VI Reference In"=w486, "error in"=w485, "Acq Control.Cancel Acq"="Cancel") -> ("FPGA VI Reference Out"=w484:refnum<k20>, "error out"=w483:errorcluster, "Acq Status.Acq In Progress"=w482:bool, "Acq Status.Frames Acq'd"=w481:u32)
            n128 = Greater?(x=w481, y=w489) -> (0:w487:bool)
            n129 = Compound Arithmetic op=OR(invert w482, w487) -> (w488:bool)
          }
          n130 = case shown="False" w446 {
            tunnel: w445 -> [w468 w479]
            tunnel: [w463 w478] -> w456
            tunnel: w453 -> [w470 w477]
            tunnel: w452 -> [w469 w476]
            tunnel: [w457 w475] -> w451
            tunnel: w450 -> [w458 w474]
            tunnel: [w462 w473] -> w449
            tunnel: [_ w472] -> w448
            tunnel: [w468 w471] -> w447
            tunnel: w443 -> [w467 _]
            frame False {
              n131 = xnode "Read/Write Control"("FPGA VI Reference In"=w469, "error in"=w470, "Acq Control.Line Scan Height"=w467, "Acq Control.Frames To Acq"=u32 0 ("Frames To Acquire")) -> ("FPGA VI Reference Out"=w465:refnum<k20>, "error out"=w464:errorcluster)
              n132 = call "Rising Edge Detect.vi"("Input"="Acquire") -> ("Pulse"=w461:bool)  [unwired: 4 in]
              n133 = xnode "Read/Write Control"("FPGA VI Reference In"=w465, "error in"=w464, "Acq Control.Acquire"=w461) -> ("FPGA VI Reference Out"=w463:refnum<k20>, "error out"=w462:errorcluster)
              n134 = Select(t=u32 0, s="Acquire", f=w458) -> (s? t:f=w457:u32)
            }
            frame True {
              n135 = xnode "Invoke Method"("FPGA VI Reference In"=w476, "error in"=w477, "元素数量"=w479) -> ("FPGA VI Reference Out"=w478:refnum<k20>, "error out"=w473:errorcluster, "数据"=w472:u64[], "剩余元素"=w471:u32)  [unwired: 1 in]
              n136 = Increment(x=w474) -> (x+1=w475:u32)
            }
          }
          n137 = feedback-in #1(w451) -> ()
          n138 = Less?(x=w447, y=w445) -> (x < y?=w444:bool)
        }
      }
      frame #2 {
        n139 = call <vilib>:"High Resolution Relative Seconds.vi"() -> ("relative seconds"=w490:dbl)
      }
    }
    n140 = disable-structure shown="Disabled" {
      disable-tunnel: w401 -> [w432 _]
      frame Disabled {
        "process" <- w432
      }
      frame Enabled {
      }
    }
    n141 = Not(x="reset frame") -> (.not. x?=w311:bool)
    n142 = Boolean To (0,1)(Boolean=w311) -> (0, 1=w316:i16)
    n143 = Subtract(x=w321, y=w320) -> (x-y=w317:dbl)
    n144 = feedback #2(-inf) -> (w319:dbl)
    n145 = Max & Min(x=w317, y=w319) -> (max(x,y)=w314:dbl)  [unwired: 1 out]
    n146 = Multiply(x=w314, y=w316) -> (x*y=w313:dbl)
    n147 = feedback-in #2(w313) -> ()
    n148 = case shown="True" w311 {
      tunnel: w314 -> [_ w434]
      tunnel: [0.0 w434] -> w310
      frame False {
      }
      frame True {
      }
    }
    "max load a frame" <- w310
    n149 = flat-sequence {
      tunnel: w397 -> [w512]
      tunnel: w406 -> [w513]
      tunnel: w407 -> [w514]
      tunnel: w408 -> [w515]
      tunnel: w409 -> [w516]
      tunnel: w412 -> [w510]
      tunnel: w413 -> [w511]
      tunnel: w415 -> [w517]
      tunnel: w417 -> [w518]
      tunnel: w420 -> [w519]
      tunnel: w425 -> [w520]
      tunnel: w393 -> [w521]
      tunnel: w430 -> [w522]
      tunnel: w431 -> [w523]
      tunnel: w322 -> [w524]
      tunnel: [w524] -> w392
      tunnel: [w523] -> w391
      tunnel: [w522] -> w390
      tunnel: [w521] -> w389
      tunnel: [w520] -> w388
      tunnel: [w519] -> w387
      tunnel: [w518] -> w386
      tunnel: [w517] -> w385
      tunnel: [w516] -> w384
      tunnel: [w515] -> w383
      tunnel: [w514] -> w382
      tunnel: [w513] -> w381
      tunnel: [w512] -> w380
      tunnel: [w509] -> w379
      tunnel: [w508] -> w378
      tunnel: [w507] -> w377
      tunnel: [w506] -> w376
      tunnel: w396 -> [w506]
      tunnel: [w505] -> w375
      tunnel: w395 -> [w505]
      tunnel: w394 -> [w504]
      tunnel: [w504] -> w374
      tunnel: w308 -> [w492]
      tunnel: [w492] -> w307
      tunnel: w306 -> [w491]
      tunnel: [w491] -> w304
      tunnel: [w569] -> w373
      tunnel: [w568] -> w372
      tunnel: [w567] -> w371
      tunnel: [w566] -> w370
      tunnel: [w565] -> w369
      tunnel: [w564] -> w368
      tunnel: [w563] -> w367
      tunnel: [w562] -> w366
      tunnel: [w544] -> w365
      tunnel: [w542] -> w364
      tunnel: [w561] -> w363
      tunnel: [w560] -> w362
      tunnel: [w559] -> w361
      tunnel: [w558] -> w360
      tunnel: [w554] -> w359
      tunnel: [w543] -> w358
      tunnel: w392 -> [w569]
      tunnel: w391 -> [w568]
      tunnel: w390 -> [w567]
      tunnel: w389 -> [w566]
      tunnel: w388 -> [w565]
      tunnel: w387 -> [w564]
      tunnel: w386 -> [w563]
      tunnel: w385 -> [w562]
      tunnel: w384 -> [w561]
      tunnel: w383 -> [w560]
      tunnel: w382 -> [w559]
      tunnel: w381 -> [w558]
      tunnel: w380 -> [w552]
      tunnel: w379 -> [w544]
      tunnel: w378 -> [w543]
      tunnel: w377 -> [w542]
      tunnel: [w541] -> w357
      tunnel: w376 -> [w541]
      tunnel: [w540] -> w356
      tunnel: w375 -> [w540]
      tunnel: [w539] -> w355
      tunnel: w374 -> [w539]
      tunnel: [w538] -> w309
      tunnel: w307 -> [w538]
      tunnel: [w537] -> w305
      tunnel: w304 -> [w537]
      tunnel: w401 -> [w621]
      tunnel: w400 -> [w620]
      tunnel: [w619] -> w399
      tunnel: w373 -> [w670]
      tunnel: w372 -> [w669]
      tunnel: w371 -> [w668]
      tunnel: w370 -> [w666]
      tunnel: w369 -> [w571]
      tunnel: w368 -> [w641]
      tunnel: w367 -> [w638]
      tunnel: w366 -> [w595]
      tunnel: w365 -> [w614]
      tunnel: w364 -> [w613]
      tunnel: w363 -> [w632]
      tunnel: w362 -> [w631]
      tunnel: w361 -> [w630]
      tunnel: w360 -> [w629]
      tunnel: w359 -> [w617]
      tunnel: [w570] -> w354
      tunnel: [w637] -> w353
      tunnel: [w614] -> w352
      tunnel: [w613] -> w351
      tunnel: [w601] -> w350
      tunnel: [w628] -> w349
      tunnel: [w627] -> w348
      tunnel: [w626] -> w347
      tunnel: [w625] -> w346
      tunnel: [w616] -> w345
      tunnel: [w615] -> w344
      tunnel: w358 -> [w602]
      tunnel: w357 -> [w611]
      tunnel: w356 -> [w609]
      tunnel: w355 -> [w604]
      tunnel: w309 -> [w584]
      tunnel: w305 -> [w583]
      tunnel: w354 -> [w916]
      tunnel: [w916] -> w343
      tunnel: w353 -> [w915]
      tunnel: [w915] -> w342
      tunnel: w352 -> [w914]
      tunnel: [w914] -> w341
      tunnel: w351 -> [w913]
      tunnel: [w913] -> w340
      tunnel: w350 -> [w912]
      tunnel: [w912] -> w339
      tunnel: w349 -> [w911]
      tunnel: [w911] -> w338
      tunnel: w348 -> [w910]
      tunnel: [w910] -> w337
      tunnel: w347 -> [w909]
      tunnel: [w909] -> w336
      tunnel: w346 -> [w908]
      tunnel: [w908] -> w335
      tunnel: w345 -> [w907]
      tunnel: [w907] -> w334
      tunnel: w344 -> [w906]
      tunnel: [w906] -> w333
      tunnel: w343 -> [w932]
      tunnel: w342 -> [w931]
      tunnel: w341 -> [w930]
      tunnel: w340 -> [w929]
      tunnel: w339 -> [w928]
      tunnel: w338 -> [w927]
      tunnel: w337 -> [w926]
      tunnel: w336 -> [w925]
      tunnel: w335 -> [w924]
      tunnel: [w923] -> w421
      tunnel: [w922] -> w422
      tunnel: w424 -> [w921]
      tunnel: w423 -> [w920]
      tunnel: w334 -> [w919]
      tunnel: w333 -> [w918]
      tunnel: [w932] -> w332
      tunnel: [w931] -> w331
      tunnel: [w930] -> w330
      tunnel: [w929] -> w329
      tunnel: [w928] -> w328
      tunnel: [w927] -> w327
      tunnel: [w926] -> w326
      tunnel: [w925] -> w325
      tunnel: [w924] -> w324
      tunnel: [w934] -> w402
      tunnel: [w935] -> w403
      tunnel: [w936] -> w404
      tunnel: [w937] -> w405
      tunnel: [w938] -> w414
      tunnel: [w939] -> w410
      tunnel: [w940] -> w411
      tunnel: [w941] -> w416
      tunnel: [w942] -> w428
      tunnel: w332 -> [w942]
      tunnel: w331 -> [w941]
      tunnel: w330 -> [w940]
      tunnel: w329 -> [w939]
      tunnel: w328 -> [w938]
      tunnel: w327 -> [w937]
      tunnel: w326 -> [w936]
      tunnel: w325 -> [w935]
      tunnel: w324 -> [w934]
      tunnel: [w933] -> w398
      frame #0 {
        n150 = stacked-sequence {
          tunnel: w511 -> [_ w534 _]
          tunnel: w510 -> [_ w533 _]
          tunnel: [_ w532 _] -> w509
          tunnel: [_ w531 _] -> w508
          tunnel: [_ w530 _] -> w507
          tunnel: [w527 _ _] -> w503
          tunnel: [_ _ w536] -> w502
          frame #0 {
            n151 = call <vilib>:"High Resolution Relative Seconds.vi"() -> ("relative seconds"=w527:dbl)
          }
          frame #1 {
            n152 = call-poly <userlib>:"DAQNavi Read.vi"("task in"=w533) -> ("data"=w529:i32, "task out"=w530:i32)  [unwired: 9 in]
            n153 = call-poly <userlib>:"DAQNavi Read.vi"("task in"=w534) -> ("data"=w535:i32, "task out"=w532:i32)  [unwired: 9 in]
            "Stage Position X" <- w535
            n154 = Negate(x=w529) -> (-x=w528:i32)
            "Stage Position Y" <- w528
            n155 = Bundle("data"=w535, w528) -> (w531:cluster{"data":i32, i32})  [unwired: 1 in]
          }
          frame #2 {
            n156 = call <vilib>:"High Resolution Relative Seconds.vi"() -> ("relative seconds"=w536:dbl)
          }
        }
        n157 = Not(x="reset position") -> (.not. x?=w495:bool)
        n158 = Boolean To (0,1)(Boolean=w495) -> (0, 1=w497:i16)
        n159 = Subtract(x=w502, y=w503) -> (x-y=w499:dbl)
        n160 = feedback #3(-inf) -> (w501:dbl)
        n161 = Max & Min(x=w499, y=w501) -> (max(x,y)=w494:dbl)  [unwired: 1 out]
        n162 = Multiply(x=w494, y=w497) -> (x*y=w496:dbl)
        n163 = feedback-in #3(w496) -> ()
        n164 = case shown="True" w495 {
          tunnel: w494 -> [_ w526]
          tunnel: [0.0 w526] -> w493
          frame False {
          }
          frame True {
          }
        }
        "max load a position" <- w493
      }
      frame #1 {
        n165 = call <vilib>:"High Resolution Relative Seconds.vi"() -> ("relative seconds"=w554:dbl)
        n166 = feedback #4() -> (w555:dbl)  [unwired: 1 in]
        n167 = feedback-in #4(w554) -> ()
        n168 = Subtract(x=w554, y=w555) -> (x-y=w557:dbl)
        "TimeDelay" <- w557
        n169 = Greater?(x=w557, y=0.0045) -> (0:w549:bool)
        n170 = Subtract(x=w554, y=w552) -> (x-y=→"time loading a frame":dbl)
        n171 = Select(t=1, s=w549, f=0) -> (s? t:f=w546:i32)
        n172 = feedback #5(0) -> (w547:i32)
        n173 = Add(x=w546, y=w547) -> (x+y=w545:i32)
        "#timeout3" <- w545
        n174 = feedback-in #5(w545) -> ()
      }
      frame #2 {
        w648 = 30.0 ("pixel/mm")
        w633 = 0.0
        w651 = T10."Map Pixel Pointer" ("Function")
        # "Convert U64 array\nto U8 array"
        # "Convert array to\nimage for display"
        n175 = disable-structure shown="Disabled" {
          disable-tunnel: w641 -> [w681 _]
          frame Disabled {
            "BKG_Global" <- w681
          }
          frame Enabled {
          }
        }
        n176 = Add(x=1, y=w638) -> (x+y=w637:u32)
        n177 = Flatten To String(anything=w666, prepend array or string size? (T)=FALSE, byte order (0:big-endian, network order)=T9."native, host order") -> (data string=w664:string)  [unwired: 1 in, 2 out]
        n178 = disable-structure shown="Disabled" {
          disable-tunnel: w637 -> [w672 _]
          frame Disabled {
            "Frame #" <- w672
          }
          frame Enabled {
          }
        }
        n179 = String To Byte Array(string=w664) -> (unsigned byte array=w663:u8[])
        n180 = call "IMAQ GetImageSize"("Image"=w641) -> ("Y Resolution"=w639:i32, "X Resolution"=w640:i32)  [unwired: 3 in, 1 out]
        n181 = Reshape Array(w663, w670, w669) -> (w667:u8[][])
        n182 = call "IMAQ ArrayToImage"("Image Pixels (U8)"=w667, "Image"=w668) -> ("Image Out"=w570:T2)  [unwired: 8 in, 1 out]
        n183 = call "IMAQ GetImagePixelPtr"("Function"=w651, "Image"=w641) -> ("LineWidth(Pixels)"=w653:i32, "Pixel Pointer out"=w654:u64)  [unwired: 4 in, 4 out]
        n184 = expression code="atan(x)"(-0.043 ("tan(theta)")) -> (w642:dbl)
        n185 = Divide(x=w648, y=10000.0) -> (x/y=w645:dbl)
        n186 = Divide(x=w648, y=12800.0) -> (x/y=w644:dbl)
        n187 = call "IMAQ GetImageSize"("Image"=w570) -> ("Y Resolution"=w605:i32, "X Resolution"=w606:i32)  [unwired: 3 in, 1 out]
        "X Resolution" <- w606
        "Y Resolution" <- w605
        n188 = call "IMAQ GetImagePixelPtr"("Function"=w651, "Image"=w570) -> ("LineWidth(Pixels)"=w658:i32, "Pixel Pointer out"=w662:u64)  [unwired: 4 in, 4 out]
        n189 = disable-structure shown="Disabled" {
          disable-tunnel: w602 -> [w671 _]
          frame Disabled {
            "Cluster" <- w671
          }
          frame Enabled {
          }
        }
        n190 = call "IMAQ SetImageSize"("Y Resolution"=w605, "X Resolution"=w606, "Image"=w571) -> ("Image Out"=w603:T2)  [unwired: 2 in, 1 out]
        n191 = Bundle(w633, w633) -> (w608:cluster{dbl, dbl})  [unwired: 1 in]
        n192 = call "IMAQ GetImagePixelPtr"("Function"=w651, "Image"=w603) -> ("LineWidth(Pixels)"=w660:i32, "Pixel Pointer out"=w661:u64)  [unwired: 4 in, 4 out]
        n193 = dll-call lib="F:/TrackingUsingOpenCV3_with_bkg_subtr_and_pred_and_temp_matching_nodisplay - 210309/fish tracking dll vc17 opencv3_4/x64/Release/fish tracking dll vc17 opencv3_4.dll" fn="?find_centroid@@YAHPEADH0H0HHHHHPEAEHHPEAV?$Point_@H@cv@@NNNHHHHHHH22PEAV?$Point_@N@2@N@Z"("ImagePtrSrc"=w662, "LineWidthSrc"=w658, "ImagePtrDst"=w661, "LineWidthDst"=w660, "ImagePtrBkg"=w654, "LineWidthBkg"=w653, "Width"=w606, "Height"=w605, "BkgWidth"=w640, "BkgHeight"=w639, "templates"=w609, "n_templates"=w611, "TemplatesSize"=48 ("Templates size"), "position"=w602, "scale_x"=w645, "scale_y"=w644, "theta"=w642, "BinThreshold"=80, "counting_threshold"=200 ("Object Threshold"), "ROI_witdth"=110, "ROI_height"=110, "width_fish"=23, "length_fish"=115, "shift"=14, "centroid_in"=w595, "centroid_out"=w595, "heading_vector"=w608, "Update_Ratio_Bkg"="update ratio") -> ("return type"=w636:i32, "centroid_out"=w601:cluster{"y":i32, "x":i32}, "heading_vector"=w600:cluster{dbl, dbl})  [unwired: 29 in, 2 out]
        "Centroid" <- w601
        "Heading" <- w600
        n194 = Quotient & Remainder(x=w621, y=2) -> (x-y*floor(x/y)=w623:i32)  [unwired: 1 out]
        n195 = Equal To 0?(x=w636) -> (x = 0?=w607:bool)
        "fish FOUND" <- w607
        n196 = Equal?(x=w623, y=0) -> (x = y?=w593:bool)
        n197 = Unbundle(w602) -> ("data"=w599:i32, w598:i32)
        n198 = Unbundle(w600) -> (w576:dbl, w575:dbl)
        n199 = Build Array(w576, w575) -> (w574:dbl[])
        n200 = call-poly <vilib>:"Array To Matrix.vi"("Real 1D Array"=w574) -> ("Real Matrix (Column Vector)"=w573:T1)
        n201 = Transpose Matrix(1:w573) -> (0:w572:T1)
        "Real Matrix 2" <- w572
        n202 = Unbundle(w601) -> ("y"=w582:i32, "x"=w581:i32)
        n203 = Build Array(w582, w581, 1) -> (w579:i32[])
        n204 = call-poly <vilib>:"Array To Matrix.vi"("Real 1D Array"=w579) -> ("Real Matrix (Column Vector)"=w578:T1)
        n205 = Transpose Matrix(1:w578) -> (0:w577:T1)
        "Real Matrix" <- w577
        n206 = call-poly <vilib>:"A x B.vi"("B"=w584, "A"=w577) -> ("A x B"=w592:T1)  [unwired: 1 out]
        "A x B" <- w592
        n207 = call-poly <vilib>:"A x B.vi"("B"=w583, "A"=w572) -> ("A x B"=w587:T1)  [unwired: 1 out]
        "A x B 2" <- w587
        n208 = call-poly <vilib>:"Matrix To Array.vi"("Real Matrix"=w592) -> ("Real 2D Array"=w591:dbl[][])
        n209 = call-poly <vilib>:"Matrix To Array.vi"("Real Matrix"=w587) -> ("Real 2D Array"=w589:dbl[][])
        n210 = Reshape Array(w591, 2) -> (w586:dbl[])
        n211 = Reshape Array(w589, 2) -> (w585:dbl[])
        n212 = Build Array (concatenate)(w599, w598, w586, w585) -> (w597:dbl[])
        n213 = case shown="True" w593 {
          tunnel: [w673 w677] -> w618
          tunnel: w604 -> [_ w679]
          tunnel: w597 -> [_ w678]
          tunnel: w570 -> [_ w675]
          frame False {
            n214 = call <vilib>:"High Resolution Relative Seconds.vi"() -> ("relative seconds"=w673:dbl)
          }
          frame True {
            n215 = call <vilib>:"High Resolution Relative Seconds.vi"() -> ("relative seconds"=w677:dbl)
            n216 = Build Array (concatenate)(w677, w678) -> (w676:dbl[])
            n217 = case shown="True" "display" {
              tunnel: w675 -> [_ w680]
              frame False {
              }
              frame True {
                "Image" <- w680
              }
            }
            n218 = Lossy Enqueue Element(queue=w679, element=w676) -> ()  [unwired: 1 in, 4 out]
          }
        }
        n219 = And(x=w607, y="Track") -> (x .and. y?=w596:bool)
        n220 = case shown="True" w596 {
          tunnel: [w693 w751] -> w616
          tunnel: [w694 w752] -> w615
          tunnel: w632 -> [w684 w818]
          tunnel: w631 -> [w691 w817]
          tunnel: w630 -> [w689 w816]
          tunnel: w582 -> [_ w737]
          tunnel: w581 -> [_ w738]
          tunnel: w576 -> [_ w808]
          tunnel: w575 -> [_ w807]
          tunnel: w629 -> [w687 w801]
          tunnel: w599 -> [_ w799]
          tunnel: w598 -> [_ w798]
          tunnel: [w685 w777] -> w628
          tunnel: [w686 w782] -> w627
          tunnel: [w690 w781] -> w626
          tunnel: [w688 w780] -> w625
          tunnel: w617 -> [_ w757]
          tunnel: w620 -> [w692 w756]
          tunnel: [w692 w755] -> w619
          tunnel: w618 -> [_ w753]
          frame False {
            n221 = event shown="[1] \"Controller\": Mouse Down" {
              selector: _ -> [_ _ _]
              dyn-events: _ -> [_ _ _]
              timeout: 1 -> [_ _ _]
              event "Controller": Mouse Up {
                n222 = event-data() -> ()  [unwired: 1 in, 8 out]
                n223 = local write "x"(0.0) -> ()
                n224 = local write "y"(0.0) -> ()
              }
              event "Controller": Mouse Down {
                n225 = event-data() -> ("Coords"=w721:T11)  [unwired: 1 in, 7 out]
                n226 = property on="Controller" class="Pict"() -> ("Position"=w720:T12, "Bounds"=w715:T13)  [unwired: 2 in, 2 out]
                n227 = Unbundle By Name(w721) -> ("Horizontal"=w719:i32, "Vertical"=w717:i32)
                n228 = Unbundle By Name(w715) -> ("Width"=w713:u32, "Height"=w709:u32)
                n229 = Unbundle By Name(w720) -> ("Left"=w718:i32, "Top"=w716:i32)
                n230 = Subtract(x=w717, y=w716) -> (x-y=w710:i32)
                n231 = Subtract(x=w719, y=w718) -> (x-y=w714:i32)
                n232 = Divide(x=w710, y=w709) -> (x/y=w702:dbl)
                n233 = Divide(x=w714, y=w713) -> (x/y=w712:dbl)
                n234 = Subtract(x=w702, y=0.5) -> (x-y=w705:dbl)
                n235 = Subtract(x=w712, y=0.5) -> (x-y=w706:dbl)
                n236 = Multiply(x=w706, y=-5.0) -> (x*y=→"x":dbl)
                n237 = Multiply(x=w705, y=5.0) -> (x*y=→"y":dbl)
              }
              event Timeout {
                n238 = event-data() -> ()  [unwired: 1 in, 3 out]
              }
            }
            n239 = Get Queue Status(queue=w684) -> (queue out=w683:refnum<queue>, max queue size=w682:i32)  [unwired: 2 in, 6 out]
            n240 = for "For循环" {
              N: w682 -> [_]
              tunnel: w683 -> [w698]
              tunnel: [w697] -> w685
              n241 = Lossy Enqueue Element(queue=w698, element=0.0) -> (queue out=w697:refnum<queue>)  [unwired: 1 in, 3 out]
            }
            n242 = Flush Queue(queue=w691) -> (queue out=w690:refnum<queue>)  [unwired: 1 in, 2 out]
            n243 = Flush Queue(queue=w689) -> (queue out=w688:refnum<queue>)  [unwired: 1 in, 2 out]
            n244 = Flush Queue(queue=w687) -> (queue out=w686:refnum<queue>)  [unwired: 1 in, 2 out]
            n245 = local read "y"() -> (w694:dbl)
            n246 = local read "x"() -> (w693:dbl)
          }
          frame True {
            w742 = 0
            w749 = 23
            w762 = 0.0
            w771 = 2
            w775 = TRUE
            w787 = 1.0
            n247 = local read "Target Y"() -> (w739:i32)
            n248 = Subtract(x=w738, y=w739) -> (x-y=w733:i32)
            n249 = Absolute Value(x=w733) -> (abs(x)=w732:i32)
            n250 = Bundle("Target X"="Target X", "Target Y"="Target Y") -> (w758:cluster{"Target X":i32, "Target Y":i32})  [unwired: 1 in]
            n251 = Greater?(x=w732, y=w749) -> (0:w747:bool)
            n252 = local read "Target X"() -> (w736:i32)
            n253 = Get Queue Status(queue=w818, return elements? (F)=w775) -> (queue out=w778:refnum<queue>, elements=w766:dbl[])  [unwired: 1 in, 6 out]
            n254 = Subtract(x=w737, y=w736) -> (x-y=w731:i32)
            n255 = Get Queue Status(queue=w817) -> (queue out=w812:refnum<queue>, max queue size=w769:i32, # elements in queue=w813:i32)  [unwired: 2 in, 5 out]
            n256 = Equal?(x=w813, y=0) -> (x = y?=w814:bool)
            n257 = Absolute Value(x=w731) -> (abs(x)=w730:i32)
            n258 = Quotient & Remainder(x=w769, y=2) -> (floor(x/y)=w767:i32)  [unwired: 1 out]
            n259 = case shown="True" w814 {
              tunnel: w812 -> [w895 w898]
              tunnel: w737 -> [w894 w899]
              tunnel: w767 -> [_ w900]
              tunnel: [w891 w897] -> w811
              tunnel: w738 -> [w893 w896]
              frame False {
                n260 = Lossy Enqueue Element(queue=w895, element=w894) -> (queue out=w892:refnum<queue>)  [unwired: 1 in, 3 out]
                n261 = Lossy Enqueue Element(queue=w892, element=w893) -> (queue out=w891:refnum<queue>)  [unwired: 1 in, 3 out]
              }
              frame True {
                n262 = for "For循环" {
                  N: w900 -> [_]
                  tunnel: w899 -> [w905]
                  tunnel: w898 -> [w904]
                  tunnel: [w901] -> w897
                  tunnel: w896 -> [w902]
                  n263 = Lossy Enqueue Element(queue=w904, element=w905) -> (queue out=w903:refnum<queue>)  [unwired: 1 in, 3 out]
                  n264 = Lossy Enqueue Element(queue=w903, element=w902) -> (queue out=w901:refnum<queue>)  [unwired: 1 in, 3 out]
                }
              }
            }
            n265 = Get Queue Status(queue=w811, return elements? (F)=w775) -> (queue out=w781:refnum<queue>, elements=w776:i32[])  [unwired: 1 in, 6 out]
            n266 = Greater?(x=w730, y=w749) -> (0:w748:bool)
            n267 = Or(x=w747, y=w748) -> (x .or. y?=w746:bool)
            n268 = Get Queue Status(queue=w816) -> (queue out=w805:refnum<queue>, max queue size=w772:i32, # elements in queue=w809:i32)  [unwired: 2 in, 5 out]
            n269 = Equal?(x=w809, y=0) -> (x = y?=w806:bool)
            n270 = Select(t=1, s=w746, f=w742) -> (s? t:f=w744:i32)
            n271 = Quotient & Remainder(x=w772, y=w771) -> (floor(x/y)=w770:i32)  [unwired: 1 out]
            n272 = case shown="True" w806 {
              tunnel: w805 -> [w880 w883]
              tunnel: w808 -> [w879 w884]
              tunnel: w770 -> [_ w885]
              tunnel: [w876 w882] -> w804
              tunnel: w807 -> [w878 w881]
              frame False {
                n273 = Lossy Enqueue Element(queue=w880, element=w879) -> (queue out=w877:refnum<queue>)  [unwired: 1 in, 3 out]
                n274 = Lossy Enqueue Element(queue=w877, element=w878) -> (queue out=w876:refnum<queue>)  [unwired: 1 in, 3 out]
              }
              frame True {
                n275 = for "For循环" {
                  N: w885 -> [_]
                  tunnel: w884 -> [w890]
                  tunnel: w883 -> [w889]
                  tunnel: [w887] -> w882
                  tunnel: w881 -> [w886]
                  n276 = Lossy Enqueue Element(queue=w889, element=w890) -> (queue out=w888:refnum<queue>)  [unwired: 1 in, 3 out]
                  n277 = Lossy Enqueue Element(queue=w888, element=w886) -> (queue out=w887:refnum<queue>)  [unwired: 1 in, 3 out]
                }
              }
            }
            n278 = Get Queue Status(queue=w804, return elements? (F)=w775) -> (queue out=w780:refnum<queue>, elements=w764:dbl[])  [unwired: 1 in, 6 out]
            n279 = local read "m(length of kernel)"() -> (w796:i32)
            n280 = local read "length of fish_history"() -> (w794:i32)
            n281 = feedback #6(w742) -> (w728:i32)
            n282 = expression code="atan(x)"(-0.043) -> (w788:dbl)
            n283 = Divide(x=1.0, y=30.0) -> (x/y=w789:dbl)
            n284 = Get Queue Status(queue=w801) -> (queue out=w800:refnum<queue>, max queue size=w774:i32, # elements in queue=w802:i32)  [unwired: 2 in, 5 out]
            n285 = Quotient & Remainder(x=w774, y=w771) -> (floor(x/y)=w773:i32)  [unwired: 1 out]
            n286 = Equal?(x=w802, y=0) -> (x = y?=w754:bool)
            n287 = case shown="True" w754 {
              tunnel: w800 -> [w865 w868]
              tunnel: w799 -> [w864 w869]
              tunnel: w773 -> [_ w870]
              tunnel: [w861 w867] -> w797
              tunnel: w798 -> [w863 w866]
              frame False {
                n288 = Lossy Enqueue Element(queue=w865, element=w864) -> (queue out=w862:refnum<queue>)  [unwired: 1 in, 3 out]
                n289 = Lossy Enqueue Element(queue=w862, element=w863) -> (queue out=w861:refnum<queue>)  [unwired: 1 in, 3 out]
              }
              frame True {
                n290 = for "For循环" {
                  N: w870 -> [_]
                  tunnel: w869 -> [w875]
                  tunnel: w868 -> [w874]
                  tunnel: [w871] -> w867
                  tunnel: w866 -> [w872]
                  n291 = Lossy Enqueue Element(queue=w874, element=w875) -> (queue out=w873:refnum<queue>)  [unwired: 1 in, 3 out]
                  n292 = Lossy Enqueue Element(queue=w873, element=w872) -> (queue out=w871:refnum<queue>)  [unwired: 1 in, 3 out]
                }
              }
            }
            n293 = Get Queue Status(queue=w797, return elements? (F)=w775) -> (queue out=w782:refnum<queue>, elements=w765:i32[])  [unwired: 1 in, 6 out]
            n294 = Max & Min(x=w730, y=w732) -> (max(x,y)=w741:i32)  [unwired: 1 out]
            n295 = Divide(x=w787, y=10000.0) -> (x/y=w784:dbl)
            n296 = Divide(x=w787, y=12800.0) -> (x/y=w783:dbl)
            n297 = feedback #7(w742) -> (w734:i32)
            n298 = case shown="True" "count" {
              tunnel: [w819 w821] -> w735
              tunnel: w734 -> [_ w820]
              tunnel: w728 -> [_ w821]
              tunnel: [w819 w820] -> w727
              frame False {
                w819 = 0
                "out of FOV 2" <- w819
                "max distance 2" <- w819
              }
              frame True {
                "out of FOV" <- w821
                "max distance" <- w820
              }
            }
            n299 = Add(x=w735, y=w744) -> (x+y=w743:i32)
            n300 = feedback-in #6(w743) -> ()
            n301 = Max & Min(x=w741, y=w727) -> (max(x,y)=w740:i32)  [unwired: 1 out]
            n302 = feedback-in #7(w740) -> ()
            n303 = Bundle(w762, w762) -> (w761:cluster{dbl, dbl})  [unwired: 1 in]
            n304 = dll-call lib="F:/TrackingUsingOpenCV3_with_bkg_subtr_and_pred_and_temp_matching_nodisplay - 210309/MPC_dll_4_vs17_cv3_4/x64/Release/MPC_dll_4_vs17_cv3_4.dll" fn="?MPC_dll@@YAHHHHNNNHNNNNNPEAV?$Point_@H@cv@@PEANPEAH21PEAV?$Point_@N@2@@Z"("m"=w796, "predict_length"=6 ("predict length"), "fish_history_length"=w794, "gammaX"=0.06, "gammaY"=0.06, "max_command"=10.0, "shift_head2yolk"=22, "scale_x"=w789, "scale_y"=w789, "theta"=w788, "scale_x2"=w784, "scale_y2"=w783, "dst_fish_position"=w758, "command_history_array"=w766, "position_history_array"=w765, "fish_tr_history_c_array"=w776, "fish_direction_history_c_array"=w764, "c0"=w761) -> ("return type"=w726:i32, "c0"=w763:cluster{dbl, dbl})  [unwired: 20 in, 2 out]
            n305 = Equal To 0?(x=w726) -> (x = 0?=w724:bool)
            n306 = Not(x=w724) -> (.not. x?=w725:bool)
            n307 = case shown="False" w725 {
              tunnel: w757 -> [w848 w860]
              tunnel: w756 -> [w847 w859]
              tunnel: [w847 w858] -> w755
              tunnel: w753 -> [w849 w857]
              frame False {
                w837 = -inf
                n308 = local read "time loading a frame"() -> (w840:dbl)
                n309 = local read "TimeDelay"() -> (w842:dbl)
                n310 = call <vilib>:"High Resolution Relative Seconds.vi"() -> ("relative seconds"=w850:dbl)
                n311 = Not(x="reset 2") -> (.not. x?=w826:bool)
                n312 = Boolean To (0,1)(Boolean=w826) -> (0, 1=w825:i16)
                n313 = Subtract(x=w850, y=w848) -> (x-y=w827:dbl)
                n314 = Subtract(x=w849, y=w848) -> (x-y=w844:dbl)
                n315 = feedback #8(w837) -> (w846:dbl)
                n316 = feedback #9(w837) -> (w843:dbl)
                n317 = feedback #10(w837) -> (w845:dbl)
                n318 = Max & Min(x=w827, y=w846) -> (max(x,y)=w836:dbl)  [unwired: 1 out]
                "max time1 detection+command" <- w836
                n319 = feedback-in #8(w836) -> ()
                n320 = Max & Min(x=w842, y=w843) -> (max(x,y)=w839:dbl)  [unwired: 1 out]
                "max time3 total" <- w839
                n321 = feedback-in #9(w839) -> ()
                n322 = Max & Min(x=w844, y=w845) -> (max(x,y)=w824:dbl)  [unwired: 1 out]
                "max time2 detection" <- w824
                n323 = Multiply(x=w824, y=w825) -> (x*y=w823:dbl)
                n324 = feedback-in #10(w823) -> ()
                n325 = Greater?(x=w827, y=0.003) -> (0:w834:bool)
                n326 = feedback #11(w837) -> (w841:dbl)
                n327 = Select(t=1, s=w834, f=0) -> (s? t:f=w831:i32)
                n328 = Max & Min(x=w840, y=w841) -> (max(x,y)=w838:dbl)  [unwired: 1 out]
                "max time4 image and position loading" <- w838
                n329 = feedback-in #11(w838) -> ()
                n330 = feedback #12(0) -> (w830:i32)
                n331 = Add(x=w831, y=w830) -> (x+y=w829:i32)
                "#timeout1" <- w829
                n332 = feedback-in #12(w829) -> ()
              }
              frame True {
                n333 = call <vilib>:"High Resolution Relative Seconds.vi"() -> ("relative seconds"=w856:dbl)
                n334 = local read "TimeDelay"() -> (w854:dbl)
                n335 = local read "time loading a frame"() -> (w851:dbl)
                n336 = Subtract(x=w856, y=w860) -> (x-y=w855:dbl)
                n337 = Subtract(x=w857, y=w860) -> (x-y=w853:dbl)
                n338 = Format Into String(initial string=w859, w855, w853, w854, w851, "\r") -> (resulting string=w858:refnum<file>)  [unwired: 2 in, 1 out]
              }
            }
            n339 = Unbundle(w763) -> (w751:dbl, w752:dbl)
            n340 = Lossy Enqueue Element(queue=w778, element=w751) -> (queue out=w779:refnum<queue>)  [unwired: 1 in, 3 out]
            n341 = Lossy Enqueue Element(queue=w779, element=w752) -> (queue out=w777:refnum<queue>)  [unwired: 1 in, 3 out]
          }
        }
      }
      frame #3 {
      }
      frame #4 {
        n342 = Negate(x=w918) -> (-x=w917:dbl)
        "电压2" <- w917
        n343 = call-poly <vilib>:"DAQmx Write.vi"("task/channels in"=w921, "data"=w919) -> ("task out"=w922:refnum<k21>)  [unwired: 11 in, 2 out]
        n344 = call-poly <vilib>:"DAQmx Write.vi"("task/channels in"=w920, "data"=w917) -> ("task out"=w923:refnum<k21>)  [unwired: 11 in, 2 out]
        "电压1" <- w919
      }
      frame #5 {
        n345 = call <vilib>:"High Resolution Relative Seconds.vi"() -> ("relative seconds"=w933:dbl)
      }
    }
    n346 = flat-sequence {
      tunnel: w312 -> [w947]
      tunnel: [w945] -> w419
      frame #0 {
        n347 = Unbundle By Name(w947) -> ("status"=w948:bool)
        n348 = local read "Stopped"() -> (w946:bool)
        n349 = Compound Arithmetic op=OR(w948, "Stop", w946) -> (w945:bool)
        n350 = local write "Stopped"(w945) -> ()
      }
    }
    n351 = feedback-in #13(w419) -> ()
    n352 = feedback #13() -> (w418:bool)  [unwired: 1 in]
    n353 = node-c288() -> ()  [unwired: 1 in, 1 out]
  }
  n354 = Close File(refnum=w30) -> ()  [unwired: 1 in, 2 out]
  n355 = call-poly <vilib>:"DAQmx Write.vi"("task/channels in"=w83, "data"=0.0) -> ("task out"=w81:refnum<k21>)  [unwired: 11 in, 2 out]
  n356 = call <vilib>:"DAQmx Stop Task.vi"("task/channels in"=w81) -> ("task out"=w77:refnum<k21>)  [unwired: 13 in, 1 out]
  n357 = call-poly <vilib>:"DAQmx Write.vi"("task/channels in"=w82, "data"=0.0) -> ("task out"=w79:refnum<k21>)  [unwired: 11 in, 2 out]
  n358 = call <vilib>:"DAQmx Stop Task.vi"("task/channels in"=w79) -> ("task out"=w76:refnum<k21>)  [unwired: 13 in, 1 out]
  n359 = call <vilib>:"DAQmx Clear Task.vi"("task in"=w77) -> ()  [unwired: 14 in, 1 out]
  n360 = call <vilib>:"DAQmx Clear Task.vi"("task in"=w76) -> ()  [unwired: 14 in, 1 out]
  n361 = node-c288(w16) -> ()  [unwired: 1 out]
  n362 = Release Queue(queue=w37) -> ()  [unwired: 2 in, 3 out]
  n363 = Release Queue(queue=w36) -> ()  [unwired: 2 in, 3 out]
  n364 = Release Queue(queue=w35) -> ()  [unwired: 2 in, 3 out]
  n365 = Release Queue(queue=w34) -> ()  [unwired: 2 in, 3 out]
  n366 = call <userlib>:"DAQNavi Stop Task.vi"("task in"=w58) -> ("task out"=w60:i32)  [unwired: 1 in, 1 out]
  n367 = Merge Errors(w116, w115) -> (w117:errorcluster)
  n368 = call <userlib>:"DAQNavi Stop Task.vi"("task in"=w57) -> ("task out"=w59:i32)  [unwired: 1 in, 1 out]
  n369 = flat-sequence {
    tunnel: w117 -> [w951]
    tunnel: [w951] -> w124
    tunnel: w123 -> [w952]
    tunnel: w9 -> [_]
    frame #0 {
      n370 = local write "Initialized"(FALSE ("Module Enabled")) -> ()
      n371 = call "IMAQ Dispose"("Image"=w952) -> ()  [unwired: 5 in, 1 out]
    }
  }
  n372 = call <userlib>:"DAQNavi Clear Task.vi"("task in"=w60) -> ()  [unwired: 2 in, 1 out]
  n373 = call <userlib>:"DAQNavi Clear Task.vi"("task in"=w59) -> ()  [unwired: 2 in, 1 out]
  n374 = xnode "关闭FPGA VI引用"("FPGA VI引用输入"=w125, "错误输入"=w124) -> ("错误输出"=w122:errorcluster)
  n375 = call <vilib>:"Simple Error Handler.vi"("error in (no error)"=w122) -> ()  [unwired: 4 in, 5 out]
